vi "Create_Object.vi"(8 "error in (no error)":errorcluster, 9 "Terminal Map in":map{string, T1}(c390), 10 "owner refnum":variant, 11 "Function in":refnum<class "Function.lvclass">) -> (0 "error out":errorcluster, 1 "Terminal Map Out":map{string, T1}(c390), 3 "Function out":refnum<class "Function.lvclass">)   [LabVIEW 2025, in "Function.lvclass"]
uses:
  Function.lvclass
  Controls/Terminal.ctl
  Node.lvclass/Node.ctl
  Node.lvclass
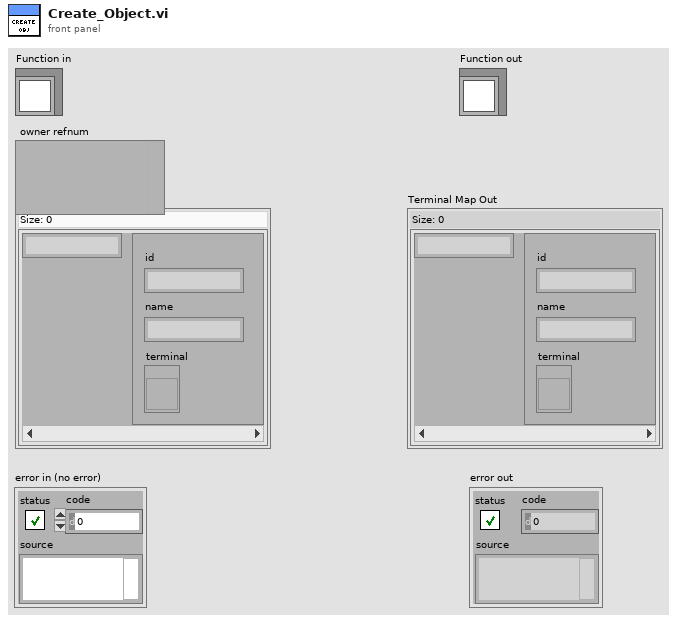
[diagram p1: front panel]
types:
  T1 = typedef "Terminal.ctl" = cluster{"id":string, "name":string, "terminal":refnum<vi>}
  T2 = typedef "LVPointTypeDef.ctl" = cluster{"Horizontal":i16, "Vertical":i16}
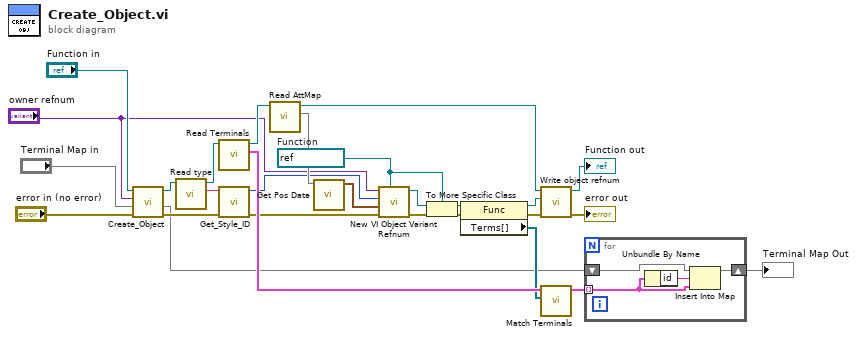
[diagram p0: block diagram]
diagram:
  w1 = refnum<vi> refnum  # Function
  n1 = call-parent "Create_Object.vi"("error in (no error)"="error in (no error)", "Terminal Map in"="Terminal Map in", "owner refnum"="owner refnum", "Node in"="Function in") -> ("error out"=w15:errorcluster, "Terminal Map Out"=w10:map{string, T1}, "Node out"=w24:refnum<class "Function.lvclass">)  [unwired: 5 in]
  n2 = call "Read type.vi"("Node in"=w24) -> ("type"=w21:string, "Node out"=w23:refnum<class "Function.lvclass">)  [unwired: 8 in, 1 out]
  n3 = call "Read Terminals.vi"("Node in"=w23) -> ("Terminals"=w17:T1[], "Node out"=w22:refnum<class "Function.lvclass">)  [unwired: 8 in, 1 out]
  n4 = call "Get_Style_ID.vi"("error in (no error)"=w15, "Style"=w21) -> ("error out"=w14:errorcluster, "style"=w13:i32)  [unwired: 7 in, 1 out]
  n5 = call "Read AttMap.vi"("Node in"=w22) -> ("AttMap"=w19:map{string, string}, "Node out"=w8:refnum<class "Function.lvclass">)  [unwired: 8 in, 1 out]
  n6 = call "Get Pos Data.vi"("AttMap"=w19) -> ("Position"=w18:T2)  [unwired: 10 in]
  n7 = call "New VI Object Variant Refnum.vi"("vi object class"=w1, "error in (no error)"=w14, "location"=w18, "style"=w13, "owner refnum"="owner refnum") -> ("error out"=w12:errorcluster, "object refnum"=w16:refnum<vi>)  [unwired: 5 in]
  n8 = To More Specific Class(target class=w1, reference=w16) -> (specific class reference=w2:refnum<vi>)  [unwired: 1 in, 1 out]
  n9 = property class="Func"(reference=w2, error in=w12) -> (reference out=w7:refnum<vi>, error out=w6:errorcluster, "Terms[]"=w11:refnum<vi>[])
  n10 = call-dynamic "Write object refnum.vi"("error in (no error)"=w6, "object refnum"=w7, "Node in"=w8) -> ("error out"=→"error out":errorcluster, "Node out"=→"Function out":refnum<class "Function.lvclass">)  [unwired: 7 in]
  n11 = call "Match Terminals.vi"("Terms[]"=w11, "Terminals"=w17) -> ("Terminals Out"=w20:T1[])  [unwired: 9 in]
  n12 = for {
    shift-right: [w30] -> w9
    shift-left: w10 -> [w31]
    tunnel: w20 -> [w29] mode=indexing
    n13 = Unbundle By Name(w29) -> ("id"=w28:string)
    n14 = Insert Into Map(map in=w31, key=w28, value=w29) -> (map out=w30:map{string, T1})  [unwired: 2 out]
  }
  "Terminal Map Out" <- w9
